vi "ValveControl.vi"() -> ()   [LabVIEW 2016]
uses:
  Classes/Controllers/I-O/Copy of NI-DAQ Folder/NI-DAQ.lvclass
panel:
  in  "CH 1 ON/OFF":bool
  in  "CH 0 ON/OFF":bool
  in  "ON/OFF":bool[](array[boolean])=[FALSE]
  in  "CH 2 ON/OFF":bool[](array[boolean])=[FALSE]
  in  "indices":i32[](array[numeric])=[0]
  in  "DAQ Module":i32
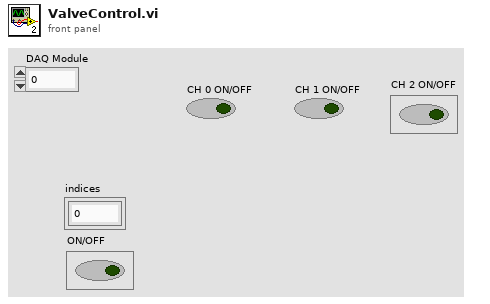
[diagram p1: front panel]
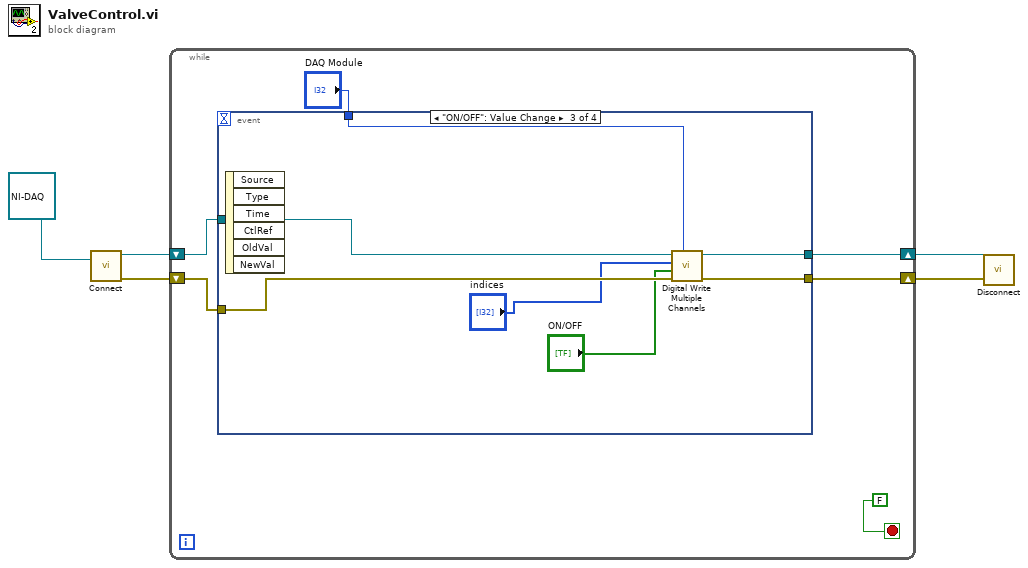
[diagram p0: block diagram]
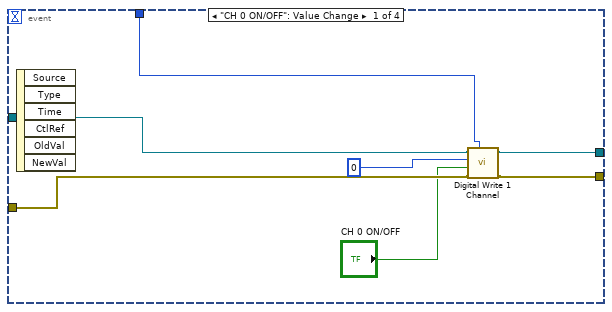
[diagram p2: hidden frame]
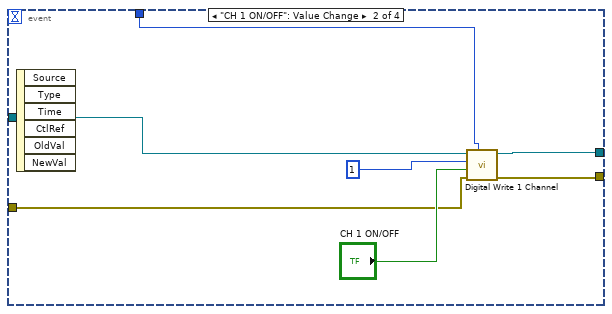
[diagram p3: hidden frame]
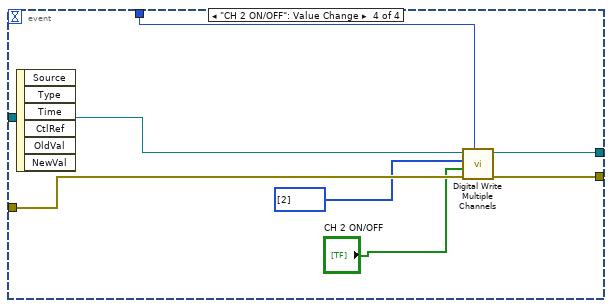
[diagram p4: hidden frame]
diagram:
  n1 = call-dynamic "Connect.vi"("NI-DAQ in"=refnum<class "NI-DAQ.lvclass"> refnum ("NI-DAQ.lvclass")) -> ("error out"=w4:errorcluster, "NI-DAQ out"=w5:refnum<class "NI-DAQ.lvclass">)  [unwired: 9 in]
  n2 = while {
    shift-right: [w9] -> w2
    shift-left: w5 -> [w11]
    shift-right: [w8] -> w1
    shift-left: w4 -> [w10]
    stop <- FALSE stop-if-true
    n3 = event shown="[2] \"ON/OFF\": Value Change" {
      selector: _ -> [_ _ _ _]
      dyn-events: _ -> [_ _ _ _]
      timeout: _ -> [_ _ _ _]
      tunnel: w11 -> [w16 w23 w32 w39]
      tunnel: w10 -> [w14 w19 w31 w38]
      tunnel: [w17 w21 w30 w37] -> w9
      tunnel: [w15 w20 w29 w36] -> w8
      tunnel: "DAQ Module" -> [w18 w22 w26 w33]
      event "CH 0 ON/OFF": Value Change {
        n4 = event-data() -> ()  [unwired: 1 in, 6 out]
        n5 = call-dynamic "Digital Write 1 Channel.vi"("DAQ Module"=w18, "error constant"=w14, "Value"="CH 0 ON/OFF", "Channel"=0, "NI-DAQ.lvclass"=w16) -> ("error IO"=w15:errorcluster, "NI-DAQ.lvclass 2"=w17:refnum<class "NI-DAQ.lvclass">)  [unwired: 5 in]
      }
      event "CH 1 ON/OFF": Value Change {
        n6 = event-data() -> ()  [unwired: 1 in, 6 out]
        n7 = call-dynamic "Digital Write 1 Channel.vi"("DAQ Module"=w22, "error constant"=w19, "Value"="CH 1 ON/OFF", "Channel"=1, "NI-DAQ.lvclass"=w23) -> ("error IO"=w20:errorcluster, "NI-DAQ.lvclass 2"=w21:refnum<class "NI-DAQ.lvclass">)  [unwired: 5 in]
      }
      event "ON/OFF": Value Change {
        n8 = event-data() -> ()  [unwired: 1 in, 6 out]
        n9 = call-dynamic "Digital Write Multiple Channels.vi"("DAQ Module"=w26, "error in (no error)"=w31, "Values"="ON/OFF", "Indices"="indices", "NI-DAQ in"=w32) -> ("error out"=w29:errorcluster, "NI-DAQ out"=w30:refnum<class "NI-DAQ.lvclass">)  [unwired: 5 in]
      }
      event "CH 2 ON/OFF": Value Change {
        n10 = event-data() -> ()  [unwired: 1 in, 6 out]
        n11 = call-dynamic "Digital Write Multiple Channels.vi"("DAQ Module"=w33, "error in (no error)"=w38, "Values"="CH 2 ON/OFF", "Indices"=i32[] [2], "NI-DAQ in"=w39) -> ("error out"=w36:errorcluster, "NI-DAQ out"=w37:refnum<class "NI-DAQ.lvclass">)  [unwired: 5 in]
      }
    }
  }
  n12 = call-dynamic "Disconnect.vi"("error in (no error)"=w1, "I-O in"=w2) -> ()  [unwired: 8 in, 1 out]
